vi "Display.vi"(8 "error in (no error)":errorcluster, 10 "SubPnl":refnum<vi>, 11 "Configurator JSON Base":refnum<class "Configurator JSON Base.lvclass">) -> (0 "error out":errorcluster, 3 "Configurator JSON Base":refnum<class "Configurator JSON Base.lvclass">)   [LabVIEW 2023, in "Configurator JSON Base.lvclass"]
uses:
  Configurator JSON Base.lvclass
panel:
  in  "Instr Configuration":string
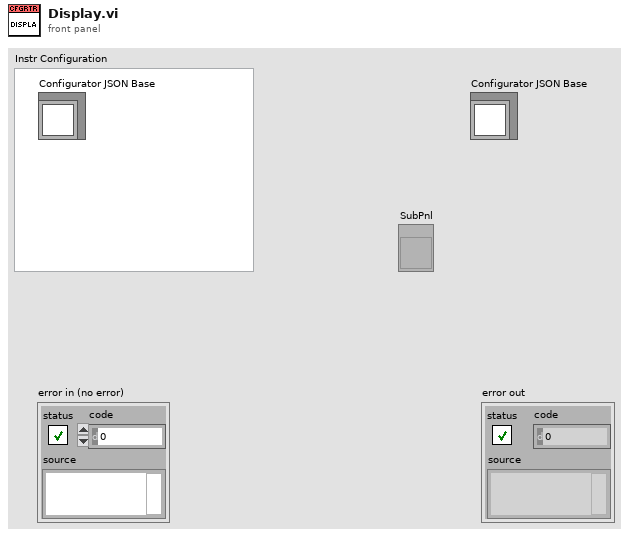
[diagram p1: front panel]
types:
  T1 = enum32{"Invalid", "Standard", "Closed", "Hidden", "Minimized", "Maximized"}
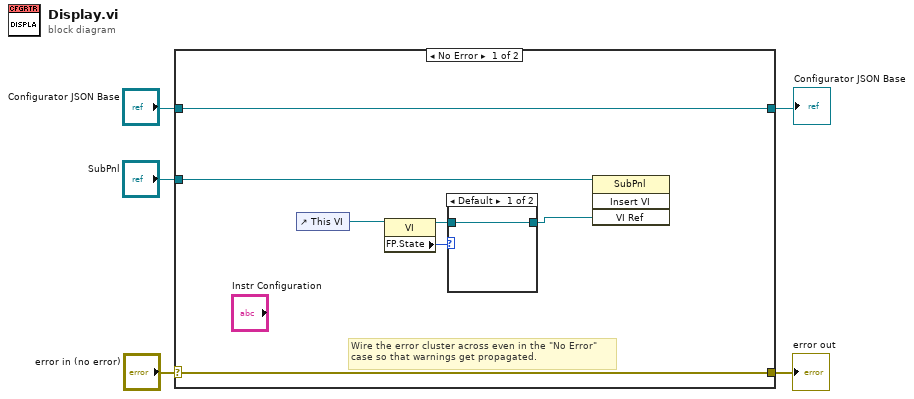
[diagram p0: block diagram]
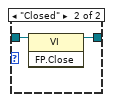
[diagram p2: hidden frame]
diagram:
  n1 = case shown="No Error" "error in (no error)" {
    selector: "error in (no error)" -> [w11 w17]
    tunnel: [w11 w17] -> w4
    tunnel: [w12 w16] -> w1
    tunnel: "Configurator JSON Base" -> [w12 w16]
    tunnel: "SubPnl" -> [w7 _]
    frame No Error {
      # "Wire the error cluster across even in the \"No Error\"\ncase so that warnings get propagated."
      n2 = control-ref of="This VI"() -> (w10:refnum<vi>)
      n3 = property class="VI"(reference=w10) -> (reference out=w8:refnum<vi>, "FP.State"=w9:T1)  [unwired: 1 in, 1 out]
      n4 = case shown="Default" w9 {
        tunnel: w8 -> [w13 w15]
        tunnel: [w13 w14] -> w6
        frame Default {
        }
        frame "Closed" {
          n5 = invoke class="VI" method="FP.Close"(reference=w15) -> (reference out=w14:refnum<vi>)  [unwired: 2 in, 2 out]
        }
      }
      n6 = invoke class="SubPnl" method="Insert VI"(reference=w7, "VI Ref"=w6) -> ()  [unwired: 2 in, 4 out]
    }
    frame Error {
    }
  }
  "error out" <- w4
  "Configurator JSON Base" <- w1
